vi "Parse Set Delimiter Example.vi"(8 "Error In":errorcluster) -> (0 "Error Out":errorcluster)   [LabVIEW 2018, in "Tests.lvlib" / "Parser.lvlib"]
uses:
  Parser.lvlib
  src/Toolkit/Tokens/Text/Text.lvclass
  src/Toolkit/Tokens/EscapedVariable/EscapedVariable.lvclass
  src/Toolkit/Tokens/Keyable/API/Keyable.lvclass/Keyable.ctl
  src/Toolkit/Tokens/Keyable/API/Read Key.vi
  src/Toolkit/Readers/String/String.lvclass
  D:/Users/cfield/Code/Field R&D Services/Mustache/trunk/src/Toolkit/Readers/Abstract/Abstract.lvclass
  <vilib>/Utility/LVClass/Get LV Class Name.vi
  src/Toolkit/Tokens/Text/API/Read Content.vi
  <vilib>/addons/_JKI Toolkits/Caraya/classes/Assert/Assert Equal_Variant.vi
  src/Toolkit/Tokens/Keyable/API/Keyable.lvclass
  <vilib>/addons/_JKI Toolkits/Caraya/classes/Test/Test.lvclass
  src/Toolkit/Parser/Parser.lvclass
  <vilib>/addons/_JKI Toolkits/Caraya/classes/Assert/Assert.lvclass
  Tests.lvlib
  src/Toolkit/Tokens/Abstract/Abstract.lvclass
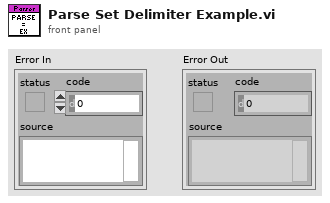
[diagram p1: front panel]
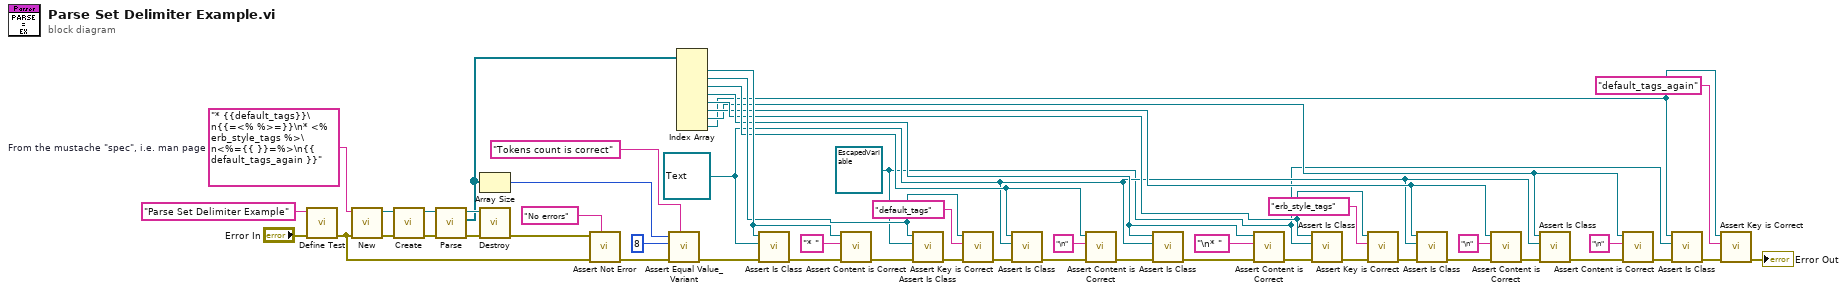
[diagram p0: block diagram]
diagram:
  w3 = refnum<class "EscapedVariable.lvclass"> refnum ("Mustache.lvlib:Tokens.lvlib:EscapedVariable.lvclass")
  w9 = refnum<class "Text.lvclass"> refnum ("Mustache.lvlib:Tokens.lvlib:Text.lvclass")
  w36 = "* {{default_tags}}\n{{=<% %>=}}\n* <% erb_style_tags %>\n<%={{ }}=%>\n{{ default_tags_again }}"  # From the mustache "spec", i.e. man page
  n1 = call <vilib>:"Define Test.vi"("error in (no error)"="Error In", "Label (VI Title)"="Parse Set Delimiter Example") -> ("error out"=w43:errorcluster)  [unwired: 9 in]
  n2 = call "New.vi"("Error In"=w43, "String"=w36) -> ("Error Out"=w49:errorcluster, "String"=w50:refnum<class "String.lvclass">)  [unwired: 8 in]
  n3 = call "Create.vi"("Error In"=w49, "Reader"=w50) -> ("Error Out"=w48:errorcluster, "Parser"=w47:refnum<class "Parser.lvclass">)  [unwired: 8 in]
  n4 = call "Parse.vi"("Error In"=w48, "Parser In"=w47) -> ("Error Out"=w45:errorcluster, "Tokens"=w37:refnum<class "Abstract.lvclass">[], "Parser Out"=w46:refnum<class "Parser.lvclass">)  [unwired: 7 in]
  n5 = Array Size(array=w37) -> (size(s)=w39:i32)
  n6 = call "Destroy.vi"("Error In"=w45, "Parser"=w46) -> ("Error Out"=w44:errorcluster)  [unwired: 8 in, 1 out]
  n7 = call <vilib>:"Assert Not Error.vi"("Label"="No errors", "error in (no error)"=w43, "Not Error?"=w44) -> ("error out"=w41:errorcluster)  [unwired: 8 in]
  n8 = call <vilib>:"Assert Equal Value_Variant.vi"("Label"="Tokens count is correct", "error in (no error)"=w41, "Y"=8 ("size(s)"), "X"=w39) -> ("error out"=w35:errorcluster)  [unwired: 7 in]
  n9 = Index Array(array=w37) -> (element #1=w33:refnum<class "Abstract.lvclass">, element #2=w29:refnum<class "Abstract.lvclass">, element #3=w24:refnum<class "Abstract.lvclass">, element #4=w20:refnum<class "Abstract.lvclass">, element #5=w17:refnum<class "Abstract.lvclass">, element #6=w13:refnum<class "Abstract.lvclass">, element #7=w8:refnum<class "Abstract.lvclass">, element #8=w2:refnum<class "Abstract.lvclass">)  [unwired: 8 in]
  n10 = call "Assert Is Class.vi"("Error In"=w35, "Expected"=w9, "Actual"=w33) -> ("Error Out"=w34:errorcluster)  [unwired: 8 in]
  n11 = call "Assert Content is Correct.vi"("Error In"=w34, "Expected"="* ", "Token"=w33) -> ("Error Out"=w31:errorcluster)  [unwired: 8 in]
  n12 = call "Assert Is Class.vi"("Error In"=w31, "Expected"=w3, "Actual"=w29) -> ("Error Out"=w30:errorcluster)  [unwired: 8 in]
  n13 = call "Assert Key is Correct.vi"("Error In"=w30, "Expected"="default_tags", "Token"=w29) -> ("Error Out"=w27:errorcluster)  [unwired: 8 in]
  n14 = call "Assert Is Class.vi"("Error In"=w27, "Expected"=w9, "Actual"=w24) -> ("Error Out"=w26:errorcluster)  [unwired: 8 in]
  n15 = call "Assert Content is Correct.vi"("Error In"=w26, "Expected"="\n", "Token"=w24) -> ("Error Out"=w23:errorcluster)  [unwired: 8 in]
  n16 = call "Assert Is Class.vi"("Error In"=w23, "Expected"=w9, "Actual"=w20) -> ("Error Out"=w22:errorcluster)  [unwired: 8 in]
  n17 = call "Assert Content is Correct.vi"("Error In"=w22, "Expected"="\n* ", "Token"=w20) -> ("Error Out"=w19:errorcluster)  [unwired: 8 in]
  n18 = call "Assert Is Class.vi"("Error In"=w19, "Expected"=w3, "Actual"=w17) -> ("Error Out"=w18:errorcluster)  [unwired: 8 in]
  n19 = call "Assert Key is Correct.vi"("Error In"=w18, "Expected"="erb_style_tags", "Token"=w17) -> ("Error Out"=w15:errorcluster)  [unwired: 8 in]
  n20 = call "Assert Is Class.vi"("Error In"=w15, "Expected"=w9, "Actual"=w13) -> ("Error Out"=w14:errorcluster)  [unwired: 8 in]
  n21 = call "Assert Content is Correct.vi"("Error In"=w14, "Expected"="\n", "Token"=w13) -> ("Error Out"=w11:errorcluster)  [unwired: 8 in]
  n22 = call "Assert Is Class.vi"("Error In"=w11, "Expected"=w9, "Actual"=w8) -> ("Error Out"=w10:errorcluster)  [unwired: 8 in]
  n23 = call "Assert Content is Correct.vi"("Error In"=w10, "Expected"="\n", "Token"=w8) -> ("Error Out"=w6:errorcluster)  [unwired: 8 in]
  n24 = call "Assert Is Class.vi"("Error In"=w6, "Expected"=w3, "Actual"=w2) -> ("Error Out"=w5:errorcluster)  [unwired: 8 in]
  n25 = call "Assert Key is Correct.vi"("Error In"=w5, "Expected"="default_tags_again", "Token"=w2) -> ("Error Out"=→"Error Out":errorcluster)  [unwired: 8 in]
